vi "FTW-Endpoint-Multipart-Ask.vi"(0 "FTW TCP Endpoint":refnum<class "FTW-Endpoint-TCP.lvclass">, 5 "Message":T1, 7 "Read Timeout":i32=100 format="%dmsec", 9 "Write Timeout":i32 format="%dmsec", 11 "error in":errorcluster) -> (4 "FTW Endpoint out":refnum<class "FTW-Endpoint-TCP.lvclass">, 6 "Reply":T1, 8 "Read Timed out?":bool, 10 "Write Timed out?":bool, 15 "error out":errorcluster)   [LabVIEW 2013, in "FTW-Endpoint-TCP.lvclass"]
uses:
  FTW-Endpoint-TCP.lvclass
  Payload/FTW-MessagePayload.ctl
  Ether/FTW-Ether.lvclass
panel:
  # "Inputs"
  # "Outputs"
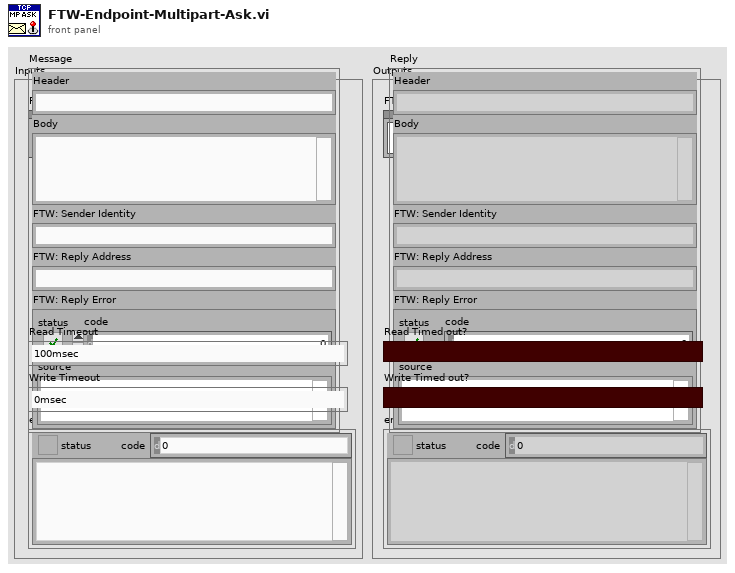
[diagram p1: front panel]
types:
  T1 = typedef "FTW-MessagePayload.ctl" = cluster{"Header":string, "Body":string, "FTW: Sender Identity":string, "FTW: Reply Address":string, "FTW: Reply Error":errorcluster}
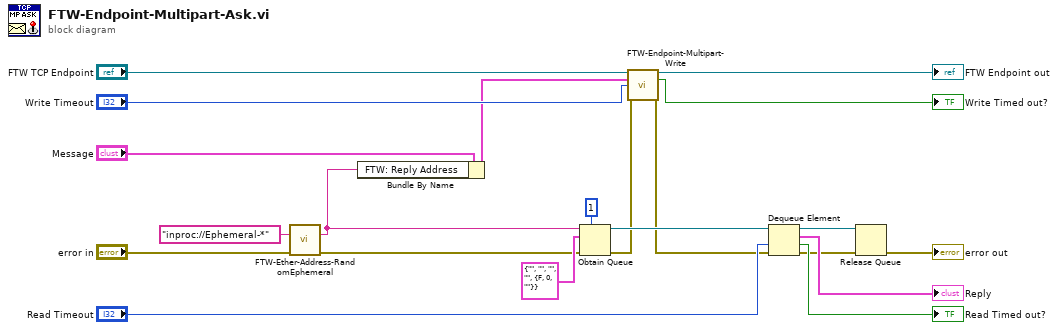
[diagram p0: block diagram]
diagram:
  n1 = call "FTW-Ether-Address-RandomEphemeral.vi"("Endpoint"="inproc://Ephemeral-*" ("Requested Ephemeral Address"), "error in"="error in") -> ("Endpoint with Replacements"=w1:string, "error out"=w3:errorcluster)  [unwired: 12 in]
  n2 = Bundle By Name(cluster="Message", "FTW: Reply Address"=w1) -> (w2:T1)
  n3 = Obtain Queue(max queue size (-1, unlimited)=1, name (unnamed)=w1, element data type=T1 {"Header"="", "Body"="", "FTW: Sender Identity"="", "FTW: Reply Address"="", "FTW: Reply Error"={"status"=FALSE, "code"=0, "source"=""}}, error in (no error)=w3) -> (queue out=w7:refnum<queue>, error out=w6:errorcluster)  [unwired: 1 in, 1 out]
  n4 = call-dynamic "FTW-Endpoint-Multipart-Write.vi"("FTW Endpoint"="FTW TCP Endpoint", "Message"=w2, "Timeout"="Write Timeout", "error in"=w6) -> ("FTW Endpoint out"=→"FTW Endpoint out":refnum<class "FTW-Endpoint-TCP.lvclass">, "Timed out?"=→"Write Timed out?":bool, "error out"=w5:errorcluster)  [unwired: 9 in]
  n5 = Dequeue Element(queue=w7, timeout in ms (-1)="Read Timeout", error in (no error)=w5) -> (queue out=w12:refnum<queue>, element=→"Reply":T1, timed out?=→"Read Timed out?":bool, error out=w11:errorcluster)
  n6 = Release Queue(queue=w12, error in (no error)=w11) -> (error out=→"error out":errorcluster)  [unwired: 1 in, 2 out]
